vi "tlc_Stop.vi"(8 "error in":errorcluster, 11 "tlc_Consumer Queue Reference.ctl":T1) -> (0 "error out":errorcluster)   [LabVIEW 2010]
uses:
  Controls/tlc_Consumer Queue Reference.ctl
  Controls/tlc_Consumer Control.ctl
  Controls/tlc_Functions.ctl
panel:
  # "Output"
  # "Input"
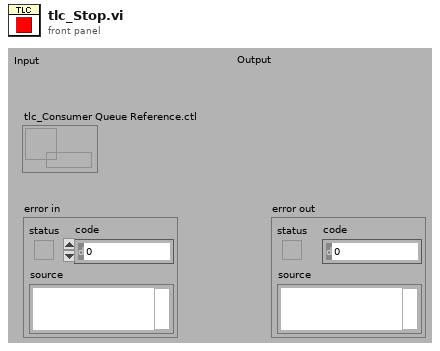
[diagram p1: front panel]
types:
  T1 = typedef "tlc_Consumer Queue Reference.ctl" = refnum<queue>
  T2 = typedef "tlc_Consumer Control.ctl" = cluster{"Command":T3, "Data":variant}
  T3 = typedef "tlc_Functions.ctl" = enum16{"Initialize", "Record", "Load", "Save", "Play", "Stop", "Exit"}
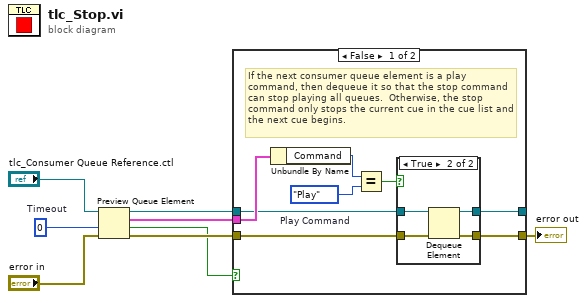
[diagram p0: block diagram]
diagram:
  w4 = 0  # Timeout
  n1 = Preview Queue Element(queue="tlc_Consumer Queue Reference.ctl", timeout in ms (-1)=w4, error in (no error)="error in") -> (queue out=w7:T1, element=w6:T2, timed out?=w5:bool, error out=w8:errorcluster)
  n2 = case shown="False" w5 {
    tunnel: w6 -> [w16 _]
    tunnel: w7 -> [w12 w24]
    tunnel: w8 -> [w11 w23]
    tunnel: [w10 w23] -> w1
    tunnel: [w9 w24] -> _
    frame False {
      w14 = tlc_Functions."Play"  # Play Command
      # "If the next consumer queue element is a play command, then dequeue it so that the stop command can stop playing all queues.  Otherwise, the stop command only stops the current cue in the cue list and the next cue begins."
      n3 = Unbundle By Name(w16) -> ("Command"=w15:T3)
      n4 = Equal?(x=w15, y=w14) -> (x = y?=w13:bool)
      n5 = case shown="True" w13 {
        tunnel: w12 -> [w18 w22]
        tunnel: w11 -> [w17 w21]
        tunnel: [w17 w20] -> w10
        tunnel: [w18 w19] -> w9
        frame False {
        }
        frame True {
          n6 = Dequeue Element(queue=w22, error in (no error)=w21) -> (queue out=w19:T1, error out=w20:errorcluster)  [unwired: 1 in, 2 out]
        }
      }
    }
    frame True {
    }
  }
  "error out" <- w1
